vi "Global Indicators.vi"() -> ()   [LabVIEW 2020]
uses:
  Traffic Signal.ctl
  Grade Gate.ctl
  PedX Signal.ctl
  Reset.ctl
  State Control.ctl
panel:
  in  "Train N/S":bool
  in  "Cycle State":T1(ring)
  in  "State Control":T2
  in  "Reset":T3
  out "Westbound":T4
  out "PedX 8":T5
  out "PedX 7":T5
  out "PedX 6":T5
  out "PedX 5":T5
  out "PedX 4":T5
  out "PedX 3":T5
  out "PedX 2":T5
  out "PedX":T5
  out "Grade Gate East":T6
  out "Grade Gate West":T6
  out "Nothbound":T4
  out "Southbound":T4
  out "Eastbound":T4
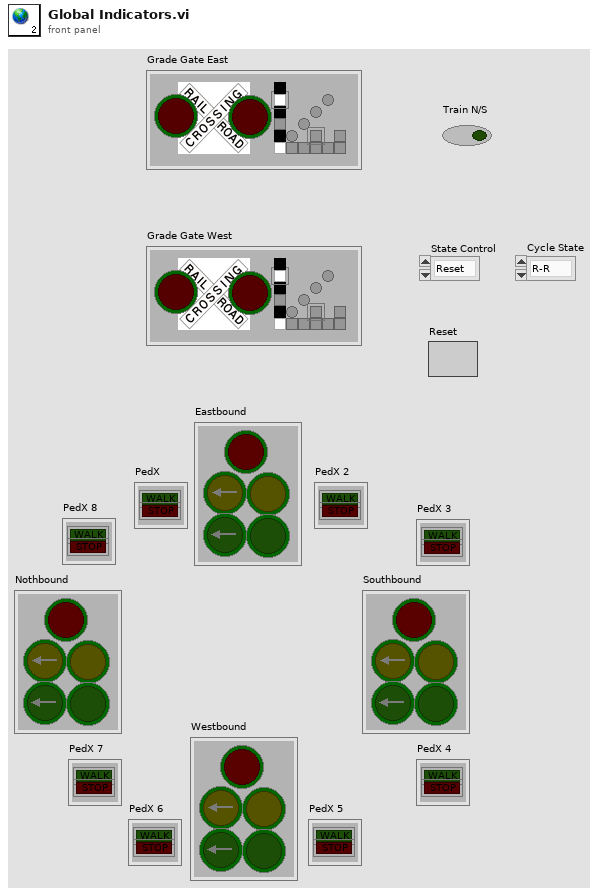
[diagram p1: front panel]
types:
  T1 = enum16{"R-R", "NS Left G", "NS Left Y", "NS Straight G", "NS Straight Y", "r-r", "WE Left G", "WE Left Y", "WE Straight G", "WE Straight Y"}
  T2 = typedef "State Control.ctl" = enum16{"Reset", "Cycle", "Train Approach"}
  T3 = typedef "Reset.ctl" = bool
  T4 = typedef "Traffic Signal.ctl" = cluster{"Red Light":bool, "Yellow Light":bool, "Green Light":bool, "Yellow Turn":bool, "Green Turn":bool}
  T5 = typedef "PedX Signal.ctl" = cluster{"PedX Walk":bool, "PedX Stop":bool}
  T6 = typedef "Grade Gate.ctl" = cluster{"UP 2":bool, "Pivot":bool, "UP 3":bool, "UP 4":bool, "UP 5":bool, "UP 6":bool, "DOWN 2":bool, "DOWN 3":bool, "DOWN 4":bool, "DOWN 5":bool, "DOWN 6":bool, "DOWN 7":bool, "DOWN 8":bool, "SIDE 2":bool, "SIDE 3":bool, "SIDE 4":bool, "SIDE 5":bool, "Blinky 2":bool, "Blinky 1":bool}
diagram:
